vi "Include Default Region in URL.vi"(11 "IAM Session":refnum<class "IAM Session.lvclass">) -> (3 "Include Default Region":bool)   [LabVIEW 2015, in "NI_AWS_IAM.lvlib" / "IAM Session.lvclass"]
uses:
  IAM Session.lvclass
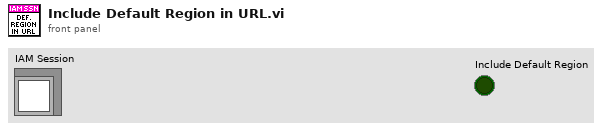
[diagram p1: front panel]
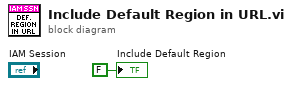
[diagram p0: block diagram]
diagram:
  "Include Default Region" <- FALSE ("Include Default Region")
